vi "decoder.vi"   [LabVIEW 2015]
uses:
  <vilib>/Erdos Miller/LV-JSON/Compose JSON String (JSON).vi
  src/lib/TOML.lvlib
  <vilib>/Erdos Miller/LV-JSON/LV-JSON.lvlib
types:
  T1 = typedef "TOML.lvlib/TOML Value.ctl" = cluster{"\\type":enum16{"Table", "Array", "String", "Integer", "Float", "Boolean", "Offset Date-Time", "Local Date-Time", "Local Date", "Local Time"}, "ÿýÿýÿýÿýÿýÿþÿýÿýÿý%LV-TOML.lvlib:TOML Key-Value Pair.ctlÿýÿýÿýÿýÿýÿþÿýÿýÿýLV-TOML.lvlib:TOML Value.ctl$":variant}
  T2 = typedef "LV-JSON.lvlib/JSON Value.ctl" = cluster{"\\type":enum16{"Object", "Array", "String", "Number", "Boolean", "Null"}, "ÿýÿýÿýÿýÿýÿþÿýÿýÿý&LV-JSON.lvlib:JSON Name-Value Pair.ctlÿýÿýÿýÿýÿýÿþÿýÿýÿýLV-JSON.lvlib:JSON Value.ctl":variant}
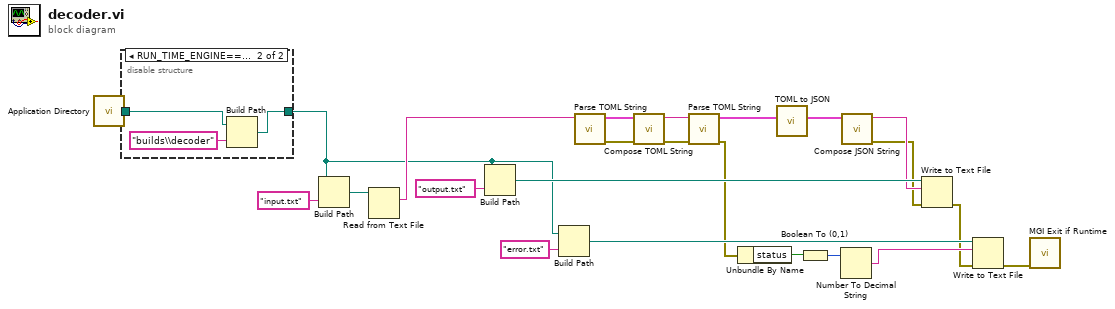
[diagram p0: block diagram]
diagram:
  n1 = call <vilib>:"Application Directory.vi"() -> ("Application Directory"=w17:path)
  n2 = disable-structure shown="RUN_TIME_ENGINE==False" {
    disable-tunnel: [w24 w26] -> w12
    disable-tunnel: w17 -> [w24 w27]
    frame condition #0 {
    }
    frame condition #1 (active) {
      n3 = Build Path(base path=w27, name or relative path="builds\\decoder") -> (appended path=w26:path)
    }
  }
  n4 = Build Path(base path=w12, name or relative path="input.txt") -> (appended path=w22:path)
  n5 = Read from Text File(file (use dialog)=w22) -> (text=w21:string)  [unwired: 3 in, 3 out]
  n6 = Build Path(base path=w12, name or relative path="output.txt") -> (appended path=w15:path)
  n7 = Build Path(base path=w12, name or relative path="error.txt") -> (appended path=w13:path)
  n8 = call "Parse TOML String.vi"("String"=w21) -> ("error out"=w6:errorcluster, "Value"=w18:T1)  [unwired: 9 in]
  n9 = call "Compose TOML String.vi"("error in (no error)"=w6, "Value"=w18) -> ("error out"=w4:errorcluster, "String"=w5:string)  [unwired: 8 in]
  n10 = call "Parse TOML String.vi"("error in (no error)"=w4, "String"=w5) -> ("error out"=w3:errorcluster, "Value"=w19:T1)  [unwired: 8 in]
  n11 = Unbundle By Name(w3) -> ("status"=w14:bool)
  n12 = call "TOML to JSON.vi"("Value"=w19) -> ("JSON Value"=w7:T2)  [unwired: 10 in]
  n13 = Boolean To (0,1)(Boolean=w14) -> (0, 1=w8:i16)
  n14 = Number To Decimal String(number=w8) -> (decimal integer string=w11:string)  [unwired: 1 in]
  n15 = call-poly <vilib>:"Compose JSON String.vi"("Value"=w7) -> ("error out"=w1:errorcluster, "String"=w2:string)  [unwired: 9 in]
  n16 = Write to Text File(file (use dialog)=w15, text=w2, error in=w1) -> (error out=w10:errorcluster)  [unwired: 1 in, 2 out]
  n17 = Write to Text File(file (use dialog)=w13, text=w11, error in=w10) -> (error out=w9:errorcluster)  [unwired: 1 in, 2 out]
  n18 = call <userlib>:"MGI Exit if Runtime.vi"("Error In (Dependency Only)"=w9) -> ()  [unwired: 11 in]
